vi "Timer_CountDown.vi"(11 "Seconds":dbl=200.0) -> ()   [LabVIEW 2015]
doc: "This VI displays the time remaining every second.\nInput parameter : the number of seconds to count down."
panel:
  out "Remaining Time":string
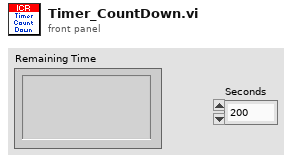
[diagram p1: front panel]
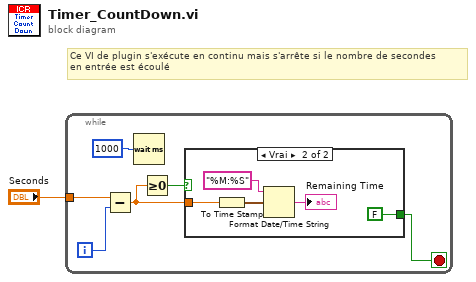
[diagram p0: block diagram]
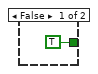
[diagram p2: hidden frame]
diagram:
  # "Ce VI de plugin s'exécute en continu mais s'arrête si le nombre de secondes\nen entrée est écoulé"
  n1 = while {
    tunnel: "Seconds" -> [w5]
    i -> [w6]
    stop <- w2 stop-if-true
    n2 = Subtract(x=w5, y=w6) -> (x-y=w3:dbl)
    n3 = Wait (ms)(milliseconds to wait=u32 1000) -> ()  [unwired: 1 out]
    n4 = Greater Or Equal To 0?(x=w3) -> (x >= 0?=w4:bool)
    n5 = case shown="Vrai" w4 {
      tunnel: w3 -> [_ w10]
      tunnel: [TRUE FALSE] -> w2
      frame False {
      }
      frame True {
        n6 = To Time Stamp(1:w10) -> (0:w12:timestamp)
        n7 = Format Date/Time String(time format string (%c)="%M:%S" ("chaîne de format de l'heure (%c)"), seconds (now)=w12) -> (date/time string=→"Remaining Time":string)  [unwired: 1 in]
      }
    }
  }
